vi "FindLines.vi"(10 "offset past match in":i32, 11 "String in":string) -> (2 "Line Number":i32, 3 "Good?":bool, 4 "Before Error":i32, 5 "Before":string, 7 "offset past match out":i32)   [LabVIEW 2016]
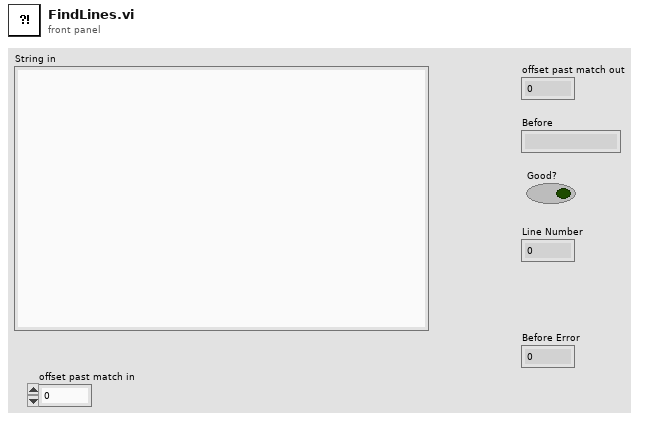
[diagram p1: front panel]
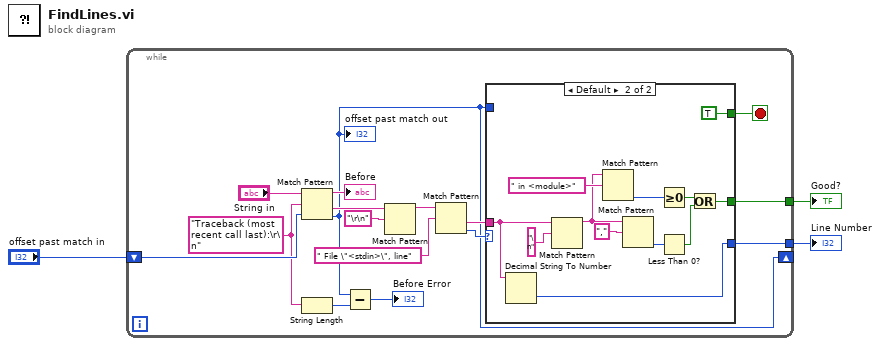
[diagram p0: block diagram]
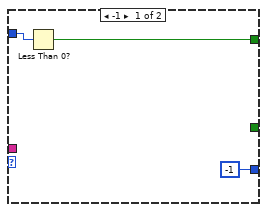
[diagram p2: hidden frame]
diagram:
  n1 = while {
    tunnel: [w19] -> w3
    tunnel: [w6] -> w1
    shift-right: [w5] -> _
    shift-left: "offset past match in" -> [w14]
    stop <- w4 stop-if-true
    w12 = "Traceback (most recent call last):\r\n"
    n2 = Match Pattern(string="String in", regular expression=w12, offset (0)=w14) -> (before substring=→"Before":string, after substring=w16:string, offset past match=w5:i32)  [unwired: 1 out]
    "offset past match out" <- w5
    n3 = String Length(string=w12) -> (length=w13:i32)
    n4 = Subtract(x=w5, y=w13) -> (x-y=→"Before Error":i32)
    n5 = Match Pattern(string=w16, regular expression="\r\n") -> (before substring=w8:string)  [unwired: 1 in, 3 out]
    n6 = Match Pattern(string=w8, regular expression=" File \"<stdin>\", line") -> (after substring=w18:string, offset past match=w7:i32)  [unwired: 1 in, 2 out]
    n7 = case shown="Default" w7 {
      tunnel: [_ w33] -> w19
      tunnel: w18 -> [_ w25]
      tunnel: [-1 w24] -> w6
      tunnel: w5 -> [w21 _]
      tunnel: [w20 TRUE] -> w4
      frame -1 {
        n8 = Less Than 0?(x=w21) -> (x < 0?=w20:bool)
      }
      frame Default {
        n9 = Decimal String To Number(string=w25) -> (number=w24:i32)  [unwired: 2 in, 1 out]
        n10 = Match Pattern(string=w25, regular expression="\n") -> (before substring=w29:string)  [unwired: 1 in, 3 out]
        n11 = Match Pattern(string=w29, regular expression=" in <module>") -> (offset past match=w30:i32)  [unwired: 1 in, 3 out]
        n12 = Match Pattern(string=w29, regular expression=",") -> (offset past match=w28:i32)  [unwired: 1 in, 3 out]
        n13 = Greater Or Equal To 0?(x=w30) -> (x >= 0?=w26:bool)
        n14 = Less Than 0?(x=w28) -> (x < 0?=w27:bool)
        n15 = Or(x=w26, y=w27) -> (x .or. y?=w33:bool)
      }
    }
  }
  "Good?" <- w3
  "Line Number" <- w1
